vi "Komponente suchen RegExp.vi"(10 "Komponente":T1, 11 "Gas":string) -> (3 "Offset nach Übereinstimmung":i32)   [LabVIEW 2020, in "System Einstellungen V2.lvlib"]
uses:
  Visualisierungs Elemente/String - Ausgabefeld.ctl
  <vilib>/regexp/Match Regular Expression.xnode
  System Einstellungen V2.lvlib
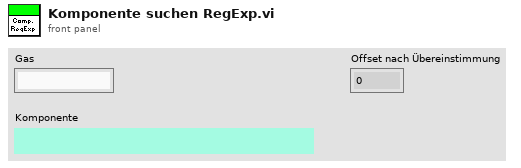
[diagram p1: front panel]
types:
  T1 = typedef "String - Ausgabefeld.ctl" = string
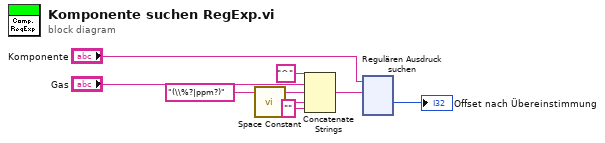
[diagram p0: block diagram]
diagram:
  n1 = call <vilib>:"Space Constant.vi"() -> ("String"=w6:string)
  n2 = Concatenate Strings("^" ("String"), "Gas", "(\\%?|ppm?)" ("String"), w6, "" ("String")) -> (w5:string)
  n3 = xnode "Regulären Ausdruck suchen"("Eingangs-String"="Komponente", "Regulärer Ausdruck"=w5) -> ("Offset nach Übereinstimmung"=→"Offset nach Übereinstimmung":i32)  [unwired: 4 in, 4 out]
